vi "getDyOfCursors.vi"(10 "error in (no error)":errorcluster, 11 "reference":refnum<vi>) -> (1 "dy":dbl, 2 "error out":errorcluster, 3 "reference out":refnum<vi>)   [LabVIEW 2014]
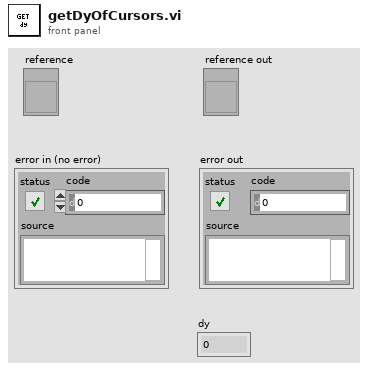
[diagram p1: front panel]
types:
  T1 = typedef "LVCursorListTypeDef.ctl" = cluster{"Name":string, "Color":u32, "Style":u8, "Point Style":u8, "Name Visible":bool, "Allow Drag":bool, "Cursor Mode":u32, "Plot":i32, "Index":i32, "Position":cluster{"X":dbl, "Y":dbl}, "X Scale":u32, "Y Scale":u32, "Watch Plots":i32[], "Watch All Plots":bool, "Plot Area":i32, "Label Offset":cluster{"X":dbl, "Y":dbl}}[]
  T2 = cluster{"Name":string, "Color":u32, "Style":u8, "Point Style":u8, "Name Visible":bool, "Allow Drag":bool, "Cursor Mode":u32, "Plot":i32, "Index":i32, "Position":cluster{"X":dbl, "Y":dbl}, "X Scale":u32, "Y Scale":u32, "Watch Plots":i32[], "Watch All Plots":bool, "Plot Area":i32, "Label Offset":cluster{"X":dbl, "Y":dbl}}
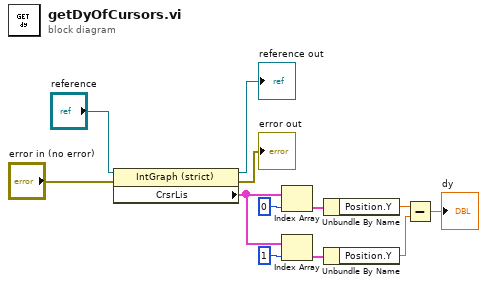
[diagram p0: block diagram]
diagram:
  n1 = property class="IntGraph (strict)"(reference="reference", error in="error in (no error)") -> (reference out=→"reference out":refnum<vi>, error out=→"error out":errorcluster, "CrsrLis"=w5:T1)
  n2 = Index Array(array=w5, index=0) -> (element=w8:T2)
  n3 = Index Array(array=w5, index=1) -> (element=w9:T2)
  n4 = Unbundle By Name(w8) -> ("Position.Y"=w10:dbl)
  n5 = Unbundle By Name(w9) -> ("Position.Y"=w11:dbl)
  n6 = Subtract(x=w10, y=w11) -> (x-y=→"dy":dbl)
